vi "getSuperKReadings.vi"(8 "error in (no error)":errorcluster, 11 "COMport":string="COM6") -> (0 "error out":errorcluster, 1 "displayInfo":u8[](array[numeric]), 2 "supplyVoltagemV":dbl, 4 "heatSinkTempC":dbl, 5 "powerReadoutPercent":u8, 6 "actualInternalTrigFreqkHz":dbl, 7 "opticalPulseFreqkHz":dbl)   [LabVIEW 2015]
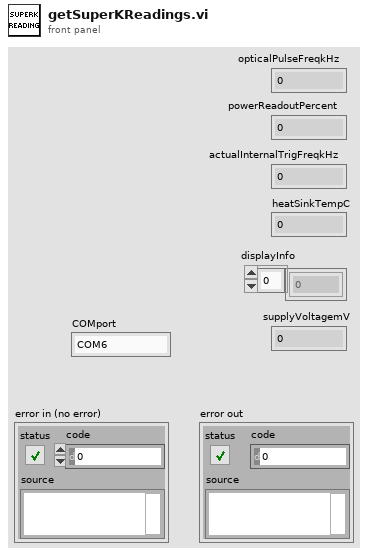
[diagram p1: front panel]
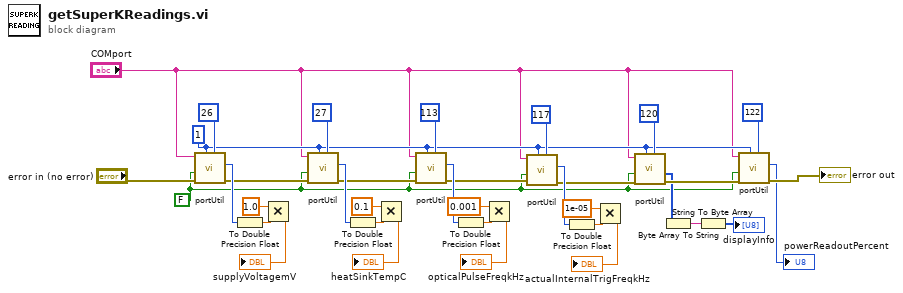
[diagram p0: block diagram]
diagram:
  w5 = FALSE ("WriteNotRead")
  w3 = u8 1 ("Destination")
  n1 = call "portUtil.vi"("Register"=u8 26, "Destination"=w3, "error in (no error)"="error in (no error)", "WriteNotRead"=w5, "COMport"="COMport") -> ("error out"=w14:errorcluster, "Long"=w33:i32)  [unwired: 4 in, 1 out]
  n2 = To Double Precision Float(number=w33) -> (double precision float=w32:dbl)
  n3 = Multiply(x=1.0, y=w32) -> (x*y=→"supplyVoltagemV":dbl)
  n4 = call "portUtil.vi"("Register"=u8 27, "Destination"=w3, "error in (no error)"=w14, "WriteNotRead"=w5, "COMport"="COMport") -> ("error out"=w13:errorcluster, "Long"=w28:i32)  [unwired: 4 in, 1 out]
  n5 = To Double Precision Float(number=w28) -> (double precision float=w27:dbl)
  n6 = Multiply(x=0.1, y=w27) -> (x*y=→"heatSinkTempC":dbl)
  n7 = call "portUtil.vi"("Register"=u8 113, "Destination"=w3, "error in (no error)"=w13, "WriteNotRead"=w5, "COMport"="COMport") -> ("error out"=w12:errorcluster, "Long"=w24:i32)  [unwired: 4 in, 1 out]
  n8 = To Double Precision Float(number=w24) -> (double precision float=w23:dbl)
  n9 = Multiply(x=0.001, y=w23) -> (x*y=→"opticalPulseFreqkHz":dbl)
  n10 = call "portUtil.vi"("Register"=u8 117, "Destination"=w3, "error in (no error)"=w12, "WriteNotRead"=w5, "COMport"="COMport") -> ("error out"=w11:errorcluster, "Long"=w19:i32)  [unwired: 4 in, 1 out]
  n11 = To Double Precision Float(number=w19) -> (double precision float=w18:dbl)
  n12 = Multiply(x=1e-05, y=w18) -> (x*y=→"actualInternalTrigFreqkHz":dbl)
  n13 = call "portUtil.vi"("Register"=u8 120, "Destination"=w3, "error in (no error)"=w11, "WriteNotRead"=w5, "COMport"="COMport") -> ("error out"=w10:errorcluster, "PayloadByteArray"=w7:u8[])  [unwired: 4 in, 1 out]
  n14 = Byte Array To String(unsigned byte array=w7) -> (string=w6:string)
  n15 = String To Byte Array(string=w6) -> (unsigned byte array=→"displayInfo":u8[])
  n16 = call "portUtil.vi"("Register"=u8 122, "Destination"=w3, "error in (no error)"=w10, "WriteNotRead"=w5, "COMport"="COMport") -> ("error out"=→"error out":errorcluster, "Long"=→"powerReadoutPercent":i32)  [unwired: 4 in, 1 out]
